vi "Drive Process.vi"   [LabVIEW 2013]
uses:
  Drive Global.vi
types:
  T1 = cluster{"Axis X":dbl, "Axis Y":dbl, "Slow Drive":bool}
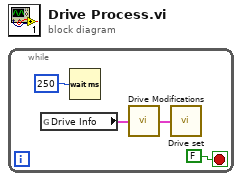
[diagram p0: block diagram]
diagram:
  n1 = while {
    stop <- FALSE stop-if-true
    n2 = global read "Drive Global.vi" "Drive Info"() -> (w2:T1)
    n3 = Wait (ms)(milliseconds to wait=u32 250) -> ()  [unwired: 1 out]
    n4 = call "Drive Modifications.vi"("Drive Info In"=w2) -> ("Drive Info Out"=w1:T1)
    n5 = call "Drive set.vi"("Drive Info In"=w1) -> ()  [unwired: 1 out]
  }
